vi "Generate Linear Accel Segment.vi"(4 "Stoopid Overlap distance":dbl min=0.0, 6 "Index":i32, 7 "Initial Acceleration":dbl format="%#_13g", 8 "Velocities":dbl[](array[numeric]), 9 "Linear Info":T2, 10 "Stoopid V":dbl=20.0, 11 "Speeds in":T1={"maxV (fps)"=20.0, "Accel Limit (fps^2)"=20.0, "Initial V (fps)"=0.0, "Sample Period (s)"=0.02, "Jerk Limit (fps^3)"=0.0, "Distances"=[]}) -> (0 "Valid":bool, 1 "Final Position":cluster{dbl, dbl, dbl}, 2 "Trajectory Segment":T3, 3 "Speeds out":T1={"maxV (fps)"=20.0, "Accel Limit (fps^2)"=20.0, "Initial V (fps)"=0.0, "Sample Period (s)"=0.02, "Jerk Limit (fps^3)"=0.0, "Distances"=[]}, 5 "Final Acceleration":dbl)   [LabVIEW 2025]
uses:
  Types/Speeds.ctl
panel:
  out "Waveform Graph":dbl[][](graph)
  out "XY Graph":cluster{dbl, dbl}[](graph)
  out "Segment Time (s)":dbl
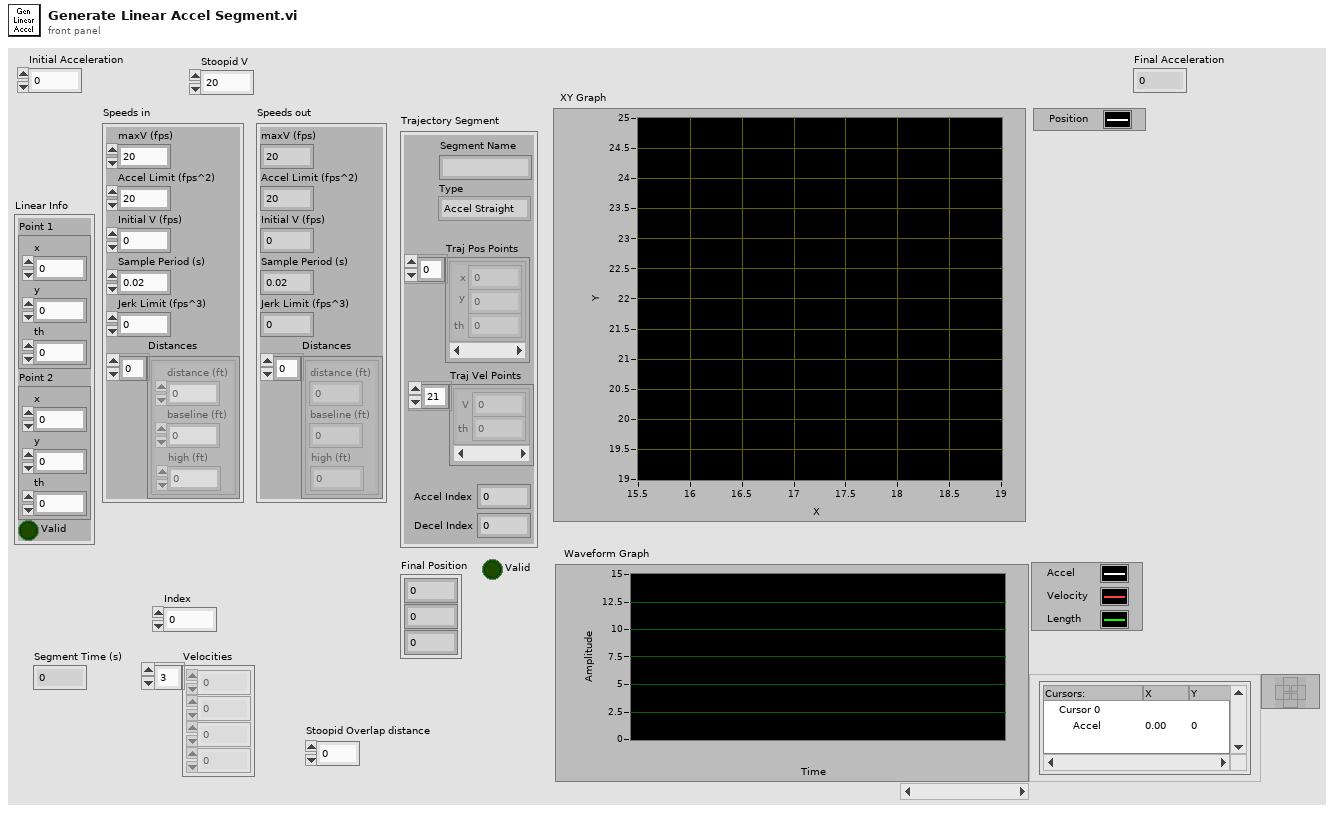
[diagram p1: front panel]
types:
  T1 = typedef "Speeds.ctl" = cluster{"maxV (fps)":dbl, "Accel Limit (fps^2)":dbl, "Initial V (fps)":dbl, "Sample Period (s)":dbl, "Jerk Limit (fps^3)":dbl, "Distances":cluster{"distance (ft)":dbl, "baseline (ft)":dbl, "high (ft)":dbl}[]}
  T2 = cluster{"Point 1":cluster{"x":dbl, "y":dbl, "th":dbl}, "Point 2":cluster{"x":dbl, "y":dbl, "th":dbl}, "Valid":bool}
  T3 = cluster{"Segment Name":string, "Type":enum16{"Accel Straight", "Const Straight", "Blend", "Circle"}, "Traj Pos Points":cluster{"x":dbl, "y":dbl, "th":dbl}[], "Traj Vel Points":cluster{"V":dbl, "th":dbl}[], "Accel Index":i32, "Decel Index":i32}
  T4 = enum16{"Accel Straight", "Const Straight", "Blend", "Circle"}
  T5 = cluster{"Accel Limit (fps^2)":dbl, "Jerk Limit (fps^3)":dbl}
  T6 = cluster{"distance (ft)":dbl, "dist baseline jerk":dbl, "dist of high Jerk":dbl}[]
  T7 = cluster{"Initial Acceleration":dbl, "Initial V (fps)":dbl}
  T8 = cluster{string, "Type":enum16{"Accel Straight", "Const Straight", "Blend", "Circle"}, cluster{dbl, dbl, dbl}[], cluster{"velocity":dbl, dbl}[], "Accel Index":i32, "Decel Index":i32}
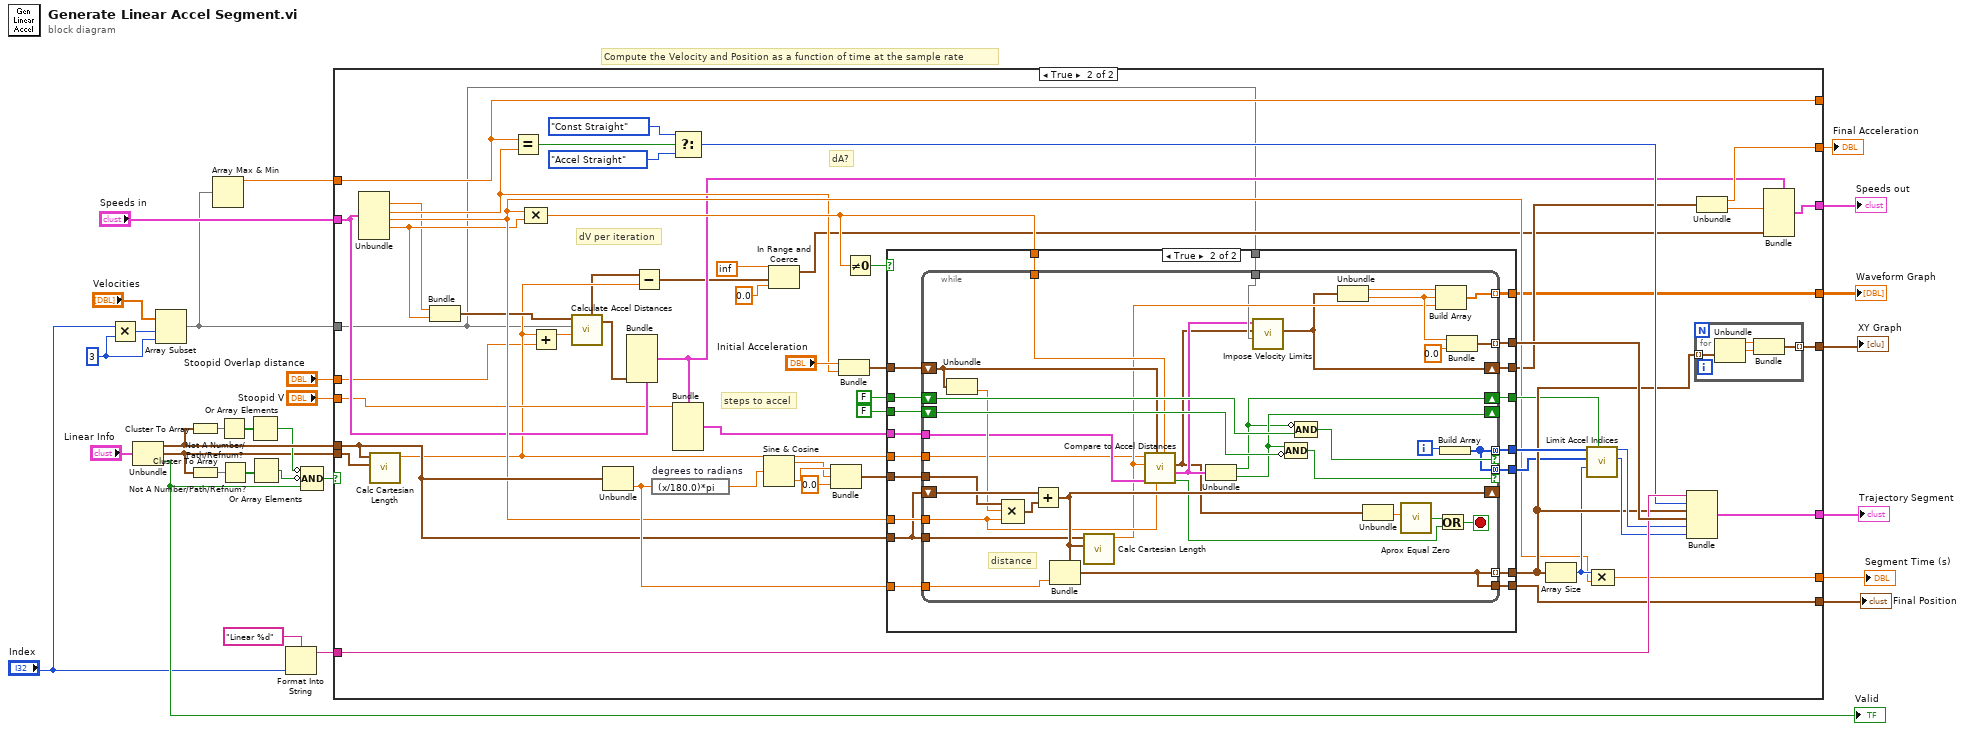
[diagram p0: block diagram]
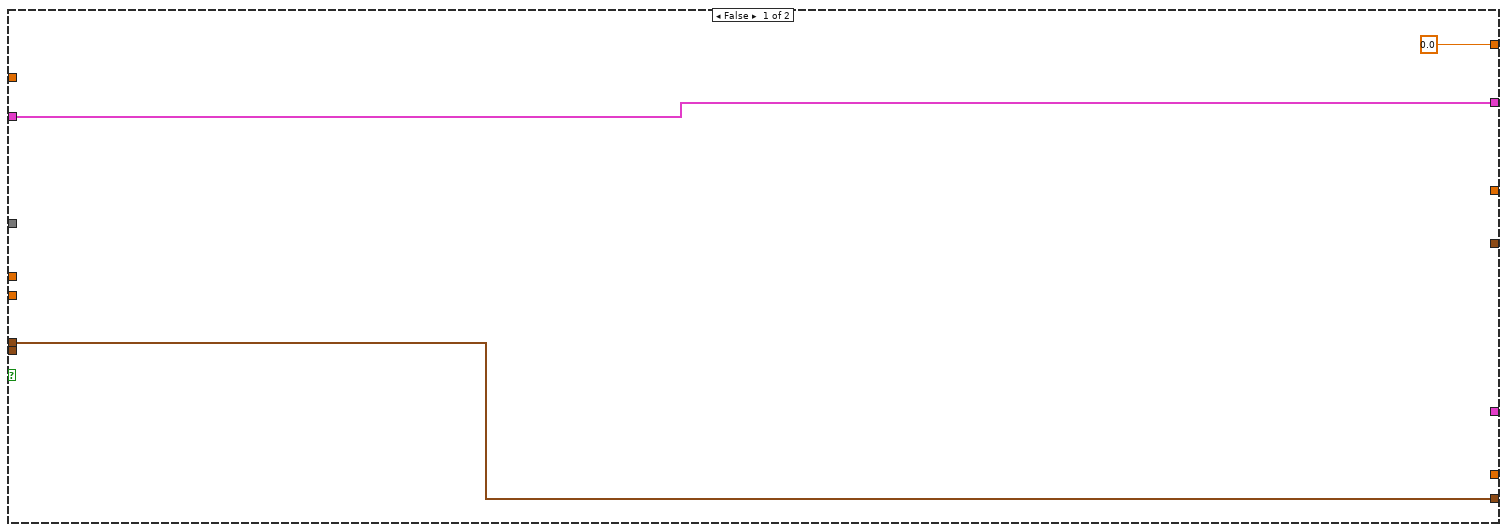
[diagram p2: hidden frame]
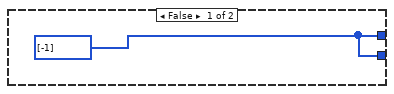
[diagram p3: hidden frame]
diagram:
  w6 = 3
  # "Compute the Velocity and Position as a function of time at the sample rate"
  n1 = Multiply(x="Index", y=w6) -> (x*y=w8:i32)
  n2 = Unbundle("Linear Info") -> ("Point 1"=w18:cluster{"x":dbl, "y":dbl, "th":dbl}, "Point 2"=w13:cluster{"x":dbl, "y":dbl, "th":dbl}, "Valid"=w19:bool)
  "Valid" <- w19
  n3 = Array Subset(array="Velocities", index=w8, length=w6) -> (w4:dbl[])
  n4 = Cluster To Array(cluster=w18) -> (array=w17:dbl[])
  n5 = Cluster To Array(cluster=w13) -> (array=w14:dbl[])
  n6 = Array Max & Min(array=w4) -> (max value=w3:dbl)  [unwired: 3 out]
  n7 = Not A Number/Path/Refnum?(number/path/refnum=w17) -> (NaN/Path/Refnum?=w16:bool[])
  n8 = Not A Number/Path/Refnum?(number/path/refnum=w14) -> (NaN/Path/Refnum?=w12:bool[])
  n9 = Or Array Elements(Boolean array=w16) -> (logical OR=w15:bool)
  n10 = Or Array Elements(Boolean array=w12) -> (logical OR=w11:bool)
  n11 = Format Into String(format string="Linear %d", "Index") -> (resulting string=w21:string)  [unwired: 2 in, 1 out]
  n12 = Compound Arithmetic op=AND(invert w15, invert w11, w19) -> (w20:bool)
  n13 = case shown="True" w20 {
    tunnel: [_ w88] -> w29
    tunnel: w21 -> [_ w82]
    tunnel: [_ w78] -> w28
    tunnel: [w31 w77] -> w27
    tunnel: [_ w74] -> w26
    tunnel: "Speeds in" -> [w32 w47]
    tunnel: [w32 w73] -> w24
    tunnel: w18 -> [w31 w68]
    tunnel: w13 -> [_ w71]
    tunnel: [_ w52] -> w10
    tunnel: [0.0 w51] -> w9
    tunnel: w4 -> [_ w33]
    tunnel: w3 -> [_ w46]
    tunnel: "Stoopid V" -> [_ w43]
    tunnel: [_ w46] -> _
    tunnel: "Stoopid Overlap distance" -> [_ w37]
    frame False {
    }
    frame True {
      # "dA?"
      # "steps to accel"
      # "dV per iteration"
      n14 = Unbundle(w47) -> ("Accel Limit (fps^2)"=w49:dbl, "Initial V (fps)"=w56:dbl, "Sample Period (s)"=w58:dbl, "Jerk Limit (fps^3)"=w50:dbl)  [unwired: 2 out]
      n15 = call "Calc Cartesian Length.vi"("Point 2"=w71, "Point 1"=w68) -> ("Length (f)"=w42:dbl)  [unwired: 8 in, 1 out]
      n16 = Bundle("Accel Limit (fps^2)"=w49, "Jerk Limit (fps^3)"=w50) -> (w48:T5)  [unwired: 1 in]
      n17 = Equal?(x=w46, y=w56) -> (x = y?=w72:bool)
      n18 = Compound Arithmetic op=MULTIPLY(w58, w50) -> (w70:dbl)
      n19 = Add(x=w42, y=w37) -> (x+y=w36:dbl)
      n20 = call "Calculate Accel Distances.vi"("Length (f)"=w36, "Velocities"=w33, "Limits"=w48) -> ("Distances"=w35:T6, "Const V Dist"=w34:T6)  [unwired: 7 in]
      n21 = Unbundle(w68) -> ("th"=w76:dbl)  [unwired: 2 out]
      n22 = Bundle(cluster=w47, "Distances"=w35) -> (w45:T1)  [unwired: 5 in]
      n23 = Subtract(x=w34, y=w42) -> (x-y=w39:T6)
      n24 = expression code="(x/180.0)*pi" "degrees to radians"(w76) -> (w75:dbl)
      n25 = Select(t=T4."Const Straight" ("Type"), s=w72, f=T4."Accel Straight" ("Type")) -> (s? t:f=w79:T4)
      n26 = Bundle(cluster=w45, "maxV (fps)"=w43) -> (w44:T1)  [unwired: 5 in]
      n27 = Sine & Cosine(0:w75) -> (1:w83:dbl, 2:w84:dbl)
      n28 = In Range and Coerce(upper limit=inf, x=w39, lower limit=0.0) -> (coerced(x)=w38:T6)  [unwired: 1 out]
      n29 = Bundle(w84, w83, 0.0) -> (w86:cluster{dbl, dbl, dbl})  [unwired: 1 in]
      n30 = Bundle("Initial Acceleration"="Initial Acceleration", "Initial V (fps)"=w56) -> (w55:T7)  [unwired: 1 in]
      n31 = Not Equal To 0?(x=w70) -> (x != 0?=w69:bool)
      n32 = case shown="True" w69 {
        tunnel: [_ w112] -> w87
        tunnel: w86 -> [_ w111]
        tunnel: [_ w110] -> w77
        tunnel: w76 -> [_ w109]
        tunnel: [_ w108] -> w62
        tunnel: [_ w107] -> w54
        tunnel: w70 -> [_ w106]
        tunnel: w58 -> [_ w105]
        tunnel: w68 -> [_ w104]
        tunnel: FALSE -> [_ w103]
        tunnel: [w93 w102] -> w65
        tunnel: w44 -> [_ w101]
        tunnel: FALSE -> [_ w100]
        tunnel: [w93 w99] -> w61
        tunnel: [_ w98] -> w59
        tunnel: w55 -> [_ w97]
        tunnel: [_ w96] -> w52
        tunnel: w42 -> [_ w95]
        tunnel: w33 -> [_ w94]
        frame False {
          w93 = i32[] [-1]
        }
        frame True {
          n33 = while {
            tunnel: [w139] -> w108 mode=indexing
            tunnel: w106 -> [w126]
            shift-right: [w113] -> w107
            shift-left: w97 -> [w129]
            tunnel: [w145] -> w112 mode=indexing
            tunnel: w105 -> [w123]
            tunnel: w111 -> [w143]
            tunnel: w109 -> [w146]
            tunnel: [w139] -> w110
            shift-right: [w141] -> _
            shift-left: w104 -> [w144]
            tunnel: w104 -> [w140]
            shift-right: [w125] -> w98
            shift-left: w103 -> [w137]
            tunnel: [w134] -> w102 mode=concatenating if=w136
            tunnel: w101 -> [w122]
            shift-right: [w128] -> _
            shift-left: w100 -> [w135]
            tunnel: [w134] -> w99 mode=concatenating if=w133
            tunnel: [w124] -> w96 mode=indexing
            tunnel: w95 -> [w118]
            tunnel: w94 -> [w116]
            i -> [w138]
            stop <- w132 stop-if-true
            # "distance"
            n34 = Unbundle(w129) -> ("Initial V (fps)"=w130:dbl)  [unwired: 1 out]
            n35 = Compound Arithmetic op=MULTIPLY(w143, w130, w123) -> (w142:cluster{dbl, dbl, dbl})
            n36 = Add(x=w144, y=w142) -> (x+y=w141:cluster{dbl, dbl, dbl})
            n37 = Bundle(cluster=w141, w146) -> (w139:cluster{dbl, dbl, dbl})  [unwired: 2 in]
            n38 = call "Calc Cartesian Length.vi"("Point 2"=w141, "Point 1"=w140) -> ("Length (f)"=w119:dbl)  [unwired: 8 in, 1 out]
            n39 = call "Compare to Accel Distances.vi"("dA"=w126, "Sample Period (s)"=w123, "Values"=w129, "Speeds in"=w122, "Current  Length"=w119, "Total Segment Length"=w118) -> ("End Loop"=w117:bool, "Ends"=w115:cluster{"Accel End":bool, "Decel End":bool}, "Values out"=w114:cluster{"accel":dbl, "velocity":dbl})  [unwired: 2 in, 1 out]
            n40 = Unbundle(w115) -> ("Accel End"=w125:bool, "Decel End"=w128:bool)
            n41 = call "Impose Velocity Limits.vi"("Array"=w116, "Values in"=w114, "Ends"=w115) -> ("Values out"=w113:cluster{"accel":dbl, "velocity":dbl})  [unwired: 8 in]
            n42 = Compound Arithmetic op=AND(w128, invert w135) -> (w133:bool)
            n43 = Compound Arithmetic op=AND(invert w125, w137) -> (w136:bool)
            n44 = Unbundle(w113) -> ("accel"=w120:dbl, "velocity"=w121:dbl)
            n45 = Unbundle(w114) -> ("velocity"=w127:dbl)  [unwired: 1 out]
            n46 = call "Aprox Equal Zero.vi"("x"=w127) -> ("Boolean"=w131:bool)  [unwired: 10 in]
            n47 = Build Array(w120, w121, w119) -> (w124:dbl[])
            n48 = Or(x=w131, y=w117) -> (x .or. y?=w132:bool)
            n49 = Build Array(w138) -> (w134:i32[])
            n50 = Bundle("velocity"=w121, 0.0) -> (w145:cluster{"velocity":dbl, dbl})  [unwired: 1 in]
          }
        }
      }
      n51 = Array Size(array=w62) -> (size(s)=w60:i32)
      n52 = call "Limit Accel Indices.vi"("Last Accel"=w59, "Size"=w60, "Decel"=w61, "Accel"=w65) -> ("Decel Index"=w64:i32, "Accel Index"=w66:i32)  [unwired: 6 in]
      n53 = Compound Arithmetic op=MULTIPLY(w60, w58) -> (w78:dbl)
      n54 = Bundle(w82, "Type"=w79, w62, w87, "Accel Index"=w66, "Decel Index"=w64) -> (w88:T8)  [unwired: 1 in]
      n55 = for {
        tunnel: w62 -> [w92] mode=indexing
        tunnel: [w89] -> w74 mode=indexing
        n56 = Unbundle(w92) -> (w91:dbl, w90:dbl)  [unwired: 1 out]
        n57 = Bundle(w91, w90) -> (w89:cluster{dbl, dbl})  [unwired: 1 in]
      }
      n58 = Unbundle(w54) -> ("Initial Acceleration"=w51:dbl, "Initial V (fps)"=w53:dbl)
      n59 = Bundle(cluster=w45, "Initial V (fps)"=w53, "Distances"=w38) -> (w73:T1)  [unwired: 4 in]
    }
  }
  "Trajectory Segment" <- w29
  "Segment Time (s)" <- w28
  "Final Position" <- w27
  "XY Graph" <- w26
  "Speeds out" <- w24
  "Waveform Graph" <- w10
  "Final Acceleration" <- w9
